vi "DirectoryExists.vi"(9 "path":string, 10 "Ftp":refnum<k24>, 11 "error in":errorcluster) -> (1 "DirectoryExists":bool, 3 "error out":errorcluster)   [LabVIEW 2015, in "UnderAutomation.Fanuc.lvlib"]
uses:
  UnderAutomation.Fanuc.lvlib
  C:/Users/fg/Documents/Fanuc.vi/LabVIEW_2024/UnderAutomation.Fanuc/lib/UnderAutomation.Fanuc.dll
  LabVIEW_2024/UnderAutomation.Fanuc/lib/UnderAutomation.Fanuc.dll
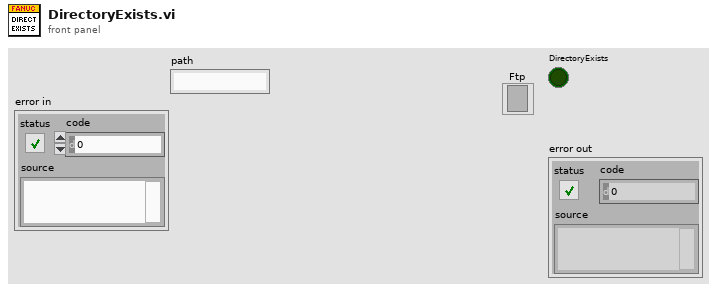
[diagram p1: front panel]
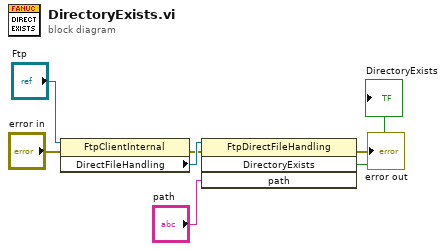
[diagram p0: block diagram]
diagram:
  n1 = property class="FtpClientInternal"(reference="Ftp", error in="error in") -> (error out=w2:errorcluster, "DirectFileHandling"=w5:refnum<k24>)  [unwired: 1 out]
  n2 = invoke class="FtpDirectFileHandling" method="DirectoryExists"(reference=w5, error in=w2, "path"="path") -> (error out=→"error out":errorcluster, "DirectoryExists"=→"DirectoryExists":bool)  [unwired: 1 in, 2 out]
